vi "DAQNavi Read (Digital Wfm 1Chan NSamp).vi"(8 "error in (no error)":errorcluster, 9 "timeout":dbl=10.0, 10 "number of samples per channel to read":u32=1000, 11 "task in":i32) -> (0 "error out":errorcluster, 2 "data":digitalwaveform(waveform)={"t0"=timestamp(0 s since 1904-01-01), "dt"=1.0, "Y"={"transitions"=[], "data"=[]}}, 3 "task out":i32)   [LabVIEW 2020]
uses:
  DAQNavi_LV.dll
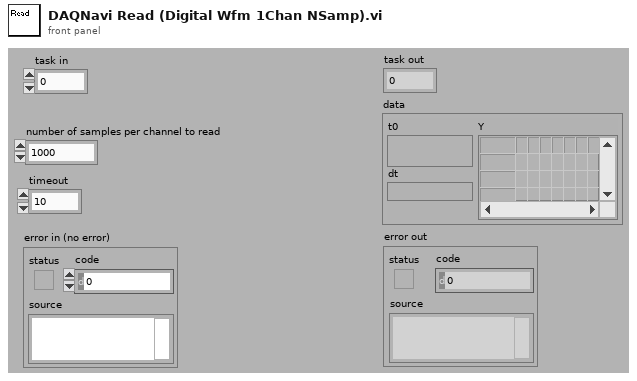
[diagram p1: front panel]
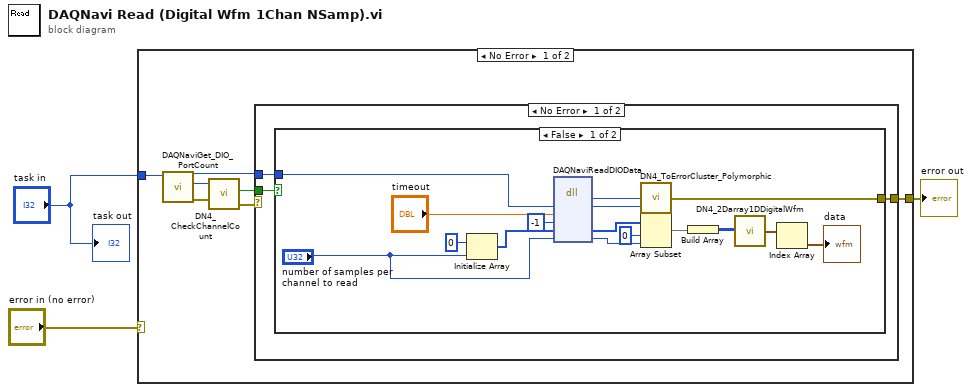
[diagram p0: block diagram]
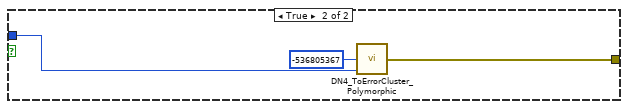
[diagram p2: hidden frame]
diagram:
  n1 = case shown="No Error" "error in (no error)" {
    selector: "error in (no error)" -> [_ w34]
    tunnel: "task in" -> [w10 _]
    tunnel: [w4 w34] -> w1
    frame No Error {
      n2 = call "DAQNaviGet_DIO_PortCount.vi"("task in"=w10) -> ("error out"=w9:errorcluster, "port count"=w8:i32, "task out"=w5:i32)  [unwired: 1 in, 7 out]
      n3 = call "DN4_CheckChannelCount.vi"("error out"=w9, "channel count"=w8) -> ("error IO"=w7:errorcluster, "greater than 1?"=w6:bool)  [unwired: 2 out]
      n4 = case shown="No Error" w7 {
        selector: w7 -> [_ w33]
        tunnel: [w13 w33] -> w4
        tunnel: w6 -> [w12 _]
        tunnel: w5 -> [w11 _]
        frame No Error {
          n5 = case shown="False" w12 {
            tunnel: [w28 w31] -> w13
            tunnel: w11 -> [w27 w30]
            frame False {
              n6 = Initialize Array(u8 0 ("element"), "number of samples per channel to read") -> (w20:u8[])
              n7 = dll-call lib="DAQNavi_LV.dll" fn="DAQNaviReadDIOData"("taskID"=w27, "timeout"="timeout", "portBit"=-1, "portData"=w20, "samples"="number of samples per channel to read") -> ("return type"=w29:i32, "taskID"=w15:i32, "portData"=w25:u8[], "samples"=w23:u32)  [unwired: 5 in, 2 out]
              n8 = call "DN4_ToErrorCluster_Polymorphic.vi"("task id"=w15, "error code"=w29) -> ("error out"=w28:errorcluster)  [unwired: 3 out]
              n9 = Array Subset(array=w25, index=0, length=w23) -> (w19:u8[])
              n10 = Build Array(w19) -> (w18:u8[][])
              n11 = call "DN4_2Darray1DDigitalWfm.vi"("data"=w18) -> ("1D Wfm"=w17:digitalwaveform[])
              n12 = Index Array(array=w17) -> (element=→"data":digitalwaveform)  [unwired: 1 in]
            }
            frame True {
              n13 = call "DN4_ToErrorCluster_Polymorphic.vi"("task id"=w30, "error code"=-536805367 ("error code (0)")) -> ("error out"=w31:errorcluster)  [unwired: 3 out]
            }
          }
        }
        frame Error {
        }
      }
    }
    frame Error {
    }
  }
  "error out" <- w1
  "task out" <- "task in"
